vi "Dynamic Class Loading.vi"() -> ()   [LabVIEW 2016]
uses:
  Source/Shared/Classes/Class Loader/Class Loader.lvclass
panel:
  out "objects":refnum<class>[](array[class])
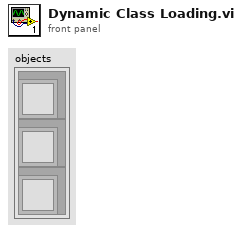
[diagram p1: front panel]
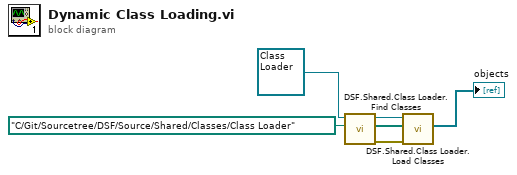
[diagram p0: block diagram]
diagram:
  n1 = call "DSF.Shared.Class Loader.Find Classes.vi"("base directory"=path "C:/Git/Sourcetree/DSF/Source/Shared/Classes/Class Loader", "Class Loader in"=refnum<class "Class Loader.lvclass"> refnum) -> ("error out"=w5:errorcluster, "class paths"=w6:path[], "Class Loader out"=w4:refnum<class "Class Loader.lvclass">)  [unwired: 7 in]
  n2 = call "DSF.Shared.Class Loader.Load Classes.vi"("error in (no error)"=w5, "class paths"=w6, "Class Loader in"=w4) -> ("objects"=→"objects":refnum<class>[])  [unwired: 6 in, 2 out]
